vi "DestroyUserEvents.vi"(8 "error in (no error)":errorcluster, 11 "Event Cluster":T1) -> (0 "error out":errorcluster)   [LabVIEW 2015]
uses:
  controls/UI Events.ctl
  User Events.lvlib
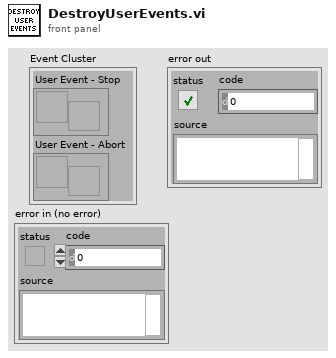
[diagram p1: front panel]
types:
  T1 = typedef "UI Events.ctl" = cluster{"User Event - Stop":refnum<user-event>, "User Event - Abort":refnum<user-event>}
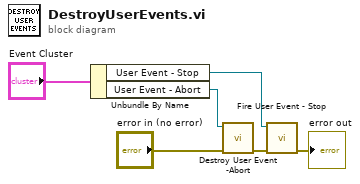
[diagram p0: block diagram]
diagram:
  n1 = Unbundle By Name("Event Cluster") -> ("User Event - Stop"=w4:refnum<user-event>, "User Event - Abort"=w5:refnum<user-event>)
  n2 = call "Destroy User Event -Abort.vi"("error in (no error)"="error in (no error)", "User Event - Abort"=w5) -> ("error out"=w6:errorcluster)  [unwired: 9 in]
  n3 = call "Fire User Event - Stop.vi"("error in (no error)"=w6, "User Event - Stop"=w4) -> ("error out"=→"error out":errorcluster)  [unwired: 9 in]
